vi "kloehn V6 - Write - Read.vi"(8 "error in":errorcluster, 10 "Send String":string, 11 "VISA Ref":refnum<visa-resource-name>) -> (0 "error out":errorcluster, 1 "Unparsed Response String":string, 2 "Parsed Response String":string, 3 "VISA Ref DUP":refnum<visa-resource-name>, 5 "Status":enum16{"Ready", "Busy"}(ring))   [LabVIEW 2010]
doc: "From user Slipknot on LV forums"
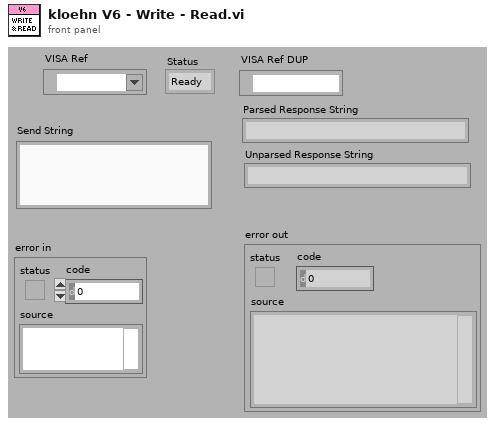
[diagram p1: front panel]
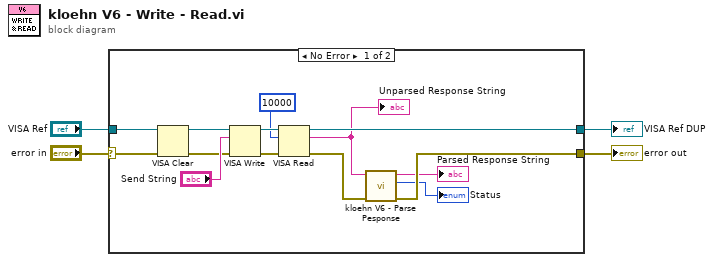
[diagram p0: block diagram]
diagram:
  n1 = case shown="No Error" "error in" {
    selector: "error in" -> [w14 w20]
    tunnel: "VISA Ref" -> [w13 w19]
    tunnel: [w7 w20] -> w3
    tunnel: [w10 w19] -> w2
    frame No Error {
      n2 = VISA Clear(VISA resource name=w13, error in (no error)=w14) -> (VISA resource name out=w11:refnum<visa-resource-name>, error out=w12:errorcluster)
      n3 = VISA Write(VISA resource name=w11, write buffer="Send String", error in (no error)=w12) -> (VISA resource name out=w17:refnum<visa-resource-name>, error out=w18:errorcluster)  [unwired: 1 out]
      n4 = VISA Read(VISA resource name=w17, byte count=u32 10000, error in (no error)=w18) -> (VISA resource name out=w10:refnum<visa-resource-name>, read buffer=w9:string, error out=w8:errorcluster)  [unwired: 1 out]
      "Unparsed Response String" <- w9
      n5 = call "kloehn V6 - Parse Pesponse.vi"("error in"=w8, "Response String"=w9) -> ("error out"=w7:errorcluster, "Status"=→"Status":enum16{"Ready", "Busy"}, "Response String"=→"Parsed Response String":string)  [unwired: 7 in]
    }
    frame Error {
    }
  }
  "VISA Ref DUP" <- w2
  "error out" <- w3
